vi "Initialize.vi"(8 "error in (no error)":errorcluster, 11 "Serial in":refnum<class "Serial.lvclass">) -> (0 "error out":errorcluster, 3 "MB_TCP out":refnum<class "Serial.lvclass">)   [LabVIEW 2021, in "Serial.lvclass"]
uses:
  Serial.lvclass
  D:/my_projects/projects/Algorithms/Labview/21/Master CR/Master CR.lvclass
  Param/TCP Param/TCP Param.lvclass
  ctl/MB timeouts.ctl
  Master CR.lvclass/Master CR.ctl
  Param/TCP Param/TCP Param.lvclass/TCP Param.ctl
  Serial.lvclass/Serial.ctl
  Master CR.lvclass
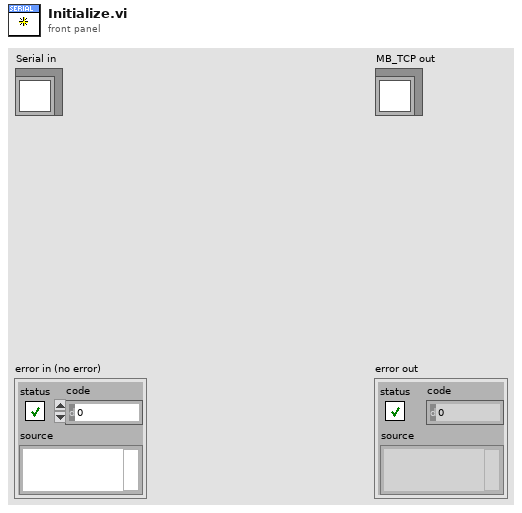
[diagram p1: front panel]
types:
  T1 = typedef "Master CR.lvclass/MB timeouts.ctl" = cluster{"reconn_timeout":i32, "N attempt max":i32, "t_reset_TTL":i32, "period":i32}
  T2 = typedef "Param.lvlib/TCP Param.lvclass/timeouts.ctl" = cluster{"conn_timeout":i32, "reconn_timeout":i32, "N attempt max":i32, "t_reset_TTL":i32, "write_timeout":i32, "read_timeout":i32, "period":i32}
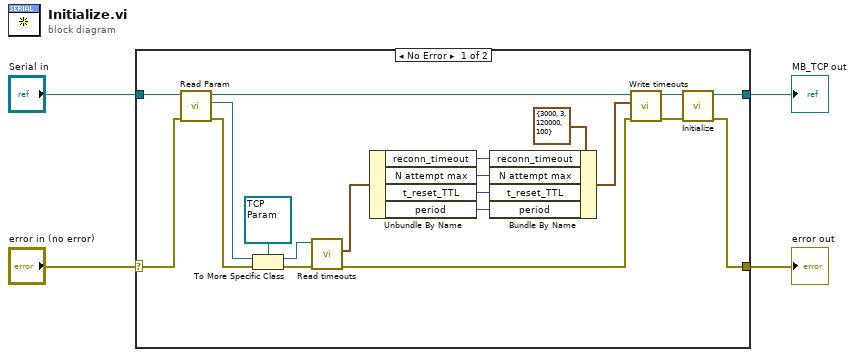
[diagram p0: block diagram]
diagram:
  n1 = case shown="No Error" "error in (no error)" {
    selector: "error in (no error)" -> [w16 w25]
    tunnel: [w9 w25] -> w1
    tunnel: [w10 w26] -> w2
    tunnel: "Serial in" -> [w13 w26]
    frame No Error {
      n2 = call "Read Param.vi"("error in (no error)"=w16, "MB_TCP in"=w13) -> ("error out"=w15:errorcluster, "Param"=w12:refnum<class "Param.lvclass">, "MB_TCP out"=w8:refnum<class "Serial.lvclass">)  [unwired: 7 in]
      n3 = To More Specific Class(target class=refnum<class "TCP Param.lvclass"> refnum ("Param.lvlib:TCP Param.lvclass"), reference=w12, error in=w15) -> (specific class reference=w14:refnum<class "TCP Param.lvclass">, error out=w23:errorcluster)
      n4 = call "Read timeouts.vi"("error in (no error)"=w23, "MBParam in"=w14) -> ("error out"=w5:errorcluster, "timeouts"=w11:T2)  [unwired: 7 in, 1 out]
      n5 = Unbundle By Name(w11) -> ("reconn_timeout"=w21:i32, "N attempt max"=w18:i32, "t_reset_TTL"=w19:i32, "period"=w20:i32)
      n6 = Bundle By Name(cluster=T1 {"reconn_timeout"=3000, "N attempt max"=3, "t_reset_TTL"=120000, "period"=100} ("MB timeouts"), "reconn_timeout"=w21, "N attempt max"=w18, "t_reset_TTL"=w19, "period"=w20) -> (w17:T1)
      n7 = call "Write timeouts.vi"("error in (no error)"=w5, "MB timeouts"=w17, "Master CR in"=w8) -> ("error out"=w6:errorcluster, "Master CR out"=w7:refnum<class "Serial.lvclass">)  [unwired: 7 in]
      n8 = call-parent "Initialize.vi"("error in (no error)"=w6, "MB in"=w7) -> ("error out"=w9:errorcluster, "MB out"=w10:refnum<class "Serial.lvclass">)  [unwired: 8 in]
    }
    frame Error {
    }
  }
  "error out" <- w1
  "MB_TCP out" <- w2
